vi "GetGlobalMenuReference.vi"(1 "Global Menu Refnum Set":refnum<k4>) -> (0 "Menu Refnum":refnum<k9>)   [LabVIEW 2012]
uses:
  GlobalMenuReference.vi
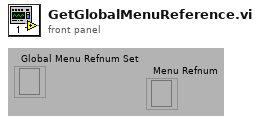
[diagram p1: front panel]
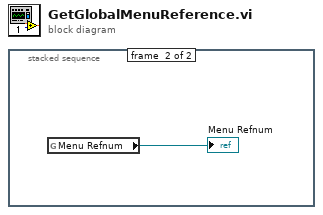
[diagram p0: block diagram]
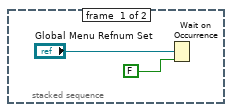
[diagram p2: hidden frame]
diagram:
  n1 = stacked-sequence {
    frame #0 {
      n2 = Wait on Occurrence(1:FALSE ("ignore previous (T)"), 2:"Global Menu Refnum Set") -> ()  [unwired: 2 out]
    }
    frame #1 {
      n3 = global read "GlobalMenuReference.vi" "Menu Refnum"() -> (→"Menu Refnum":refnum<k9>)
    }
  }
